vi "Classify Error.vi"(10 "Error Code":i32) -> (2 "Error Classification":u32)   [LabVIEW 2015, in "Tektronix 7000 Series.lvlib"]
doc: "This VI is used to check error code"
uses:
  Tektronix 7000 Series.lvlib
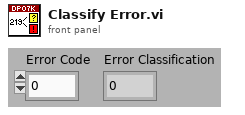
[diagram p1: front panel]
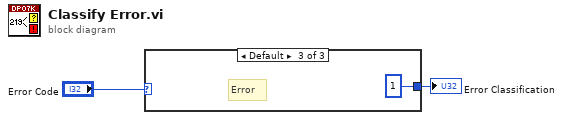
[diagram p0: block diagram]
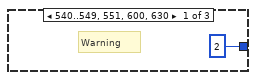
[diagram p2: hidden frame]
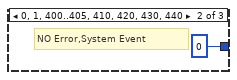
[diagram p3: hidden frame]
diagram:
  n1 = case shown="Default" "Error Code" {
    tunnel: [2 0 1] -> w1
    frame 540..549, 551, 600, 630 {
      # "Warning"
    }
    frame 0, 1, 400..405, 410, 420, 430, 440 {
      # "NO Error,System Event"
    }
    frame Default {
      # "Error"
    }
  }
  "Error Classification" <- w1
